vi "Gate Packet Words.vi"(0 "packet word in":u8[](array[numeric]), 1 "reset":bool, 5 "expected packet words":u64, 9 "input valid":bool, 12 "ready for output":bool) -> (4 "packet word out":u8[](array[numeric]), 10 "output valid out":bool, 14 "ready for input":bool)   [LabVIEW 2020, in "GettingStarted_Common_148X_FPGA.lvlib"]
uses:
  GettingStarted_Common_148X_FPGA.lvlib
  <instrlib>/_niInstr/Basic Elements/v1/FPGA/Private/Count Up U64.vi
  a7abb6bf-811a-49e6-ade6-0adeacfcc7f8.vi
  <instrlib>/_niInstr/Basic Elements/v1/FPGA/niInstr Basic Elements v1 FPGA.lvlib
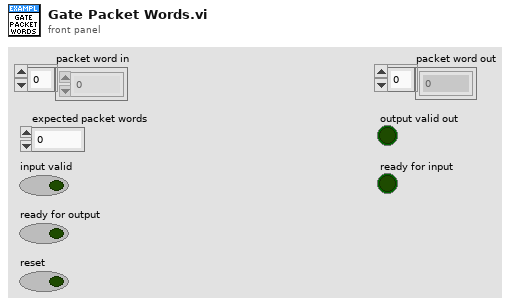
[diagram p1: front panel]
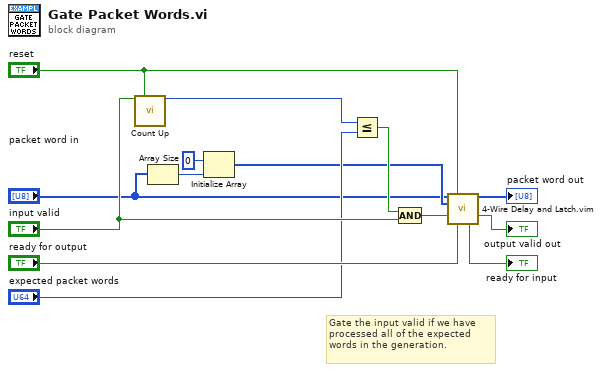
[diagram p0: block diagram]
diagram:
  # "Gate the input valid if we have processed all of the expected words in the generation."
  n1 = call-poly <instrlib>:"Count Up.vi"("increment"="input valid", "reset"="reset") -> ("count out"=w10:u64)  [unwired: 13 in]
  n2 = Array Size(array="packet word in") -> (size(s)=w4:i32)
  n3 = Initialize Array(u8 0 ("element"), w4) -> (w2:u8[])
  n4 = Less Or Equal?(x=w10, y="expected packet words") -> (x <= y?=w12:bool)
  n5 = Compound Arithmetic op=AND(w12, "input valid") -> (w8:bool)
  n6 = call "4-Wire Delay and Latch.vim"("data in"="packet word in", "reset"="reset", "default data"=w2, "input valid"=w8, "ready for output"="ready for output") -> ("data out"=→"packet word out":u8[], "output valid"=→"output valid out":bool, "ready for input"=→"ready for input":bool)  [unwired: 8 in]
